vi "Launch He Line.vi"(8 "error in (no error)":errorcluster, 9 "Interlock Chain":refnum<class "Interlock Chain.lvclass">, 11 "cRIO-CO2 in":refnum<class "cRIO-CO2.lvclass">) -> (0 "error out":errorcluster, 3 "cRIO-CO2 out":refnum<class "cRIO-CO2.lvclass">)   [LabVIEW 2015, in "cRIO-Carbondioxide.lvlib" / "cRIO-CO2.lvlib" / "cRIO-CO2.lvclass"]
uses:
  cRIO-CO2.lvclass
  Interlocks/Interlock Chain/Interlock Chain.lvclass
  He Line/He Line.lvclass
  <vilib>/ActorFramework/Actor/Actor.lvclass
  Valve/Valve.lvclass
  Valve/Action.ctl
  cRIO-CO2.lvclass/cRIO-CO2.ctl
  <vilib>/ActorFramework/Message Enqueuer/Message Enqueuer.lvclass
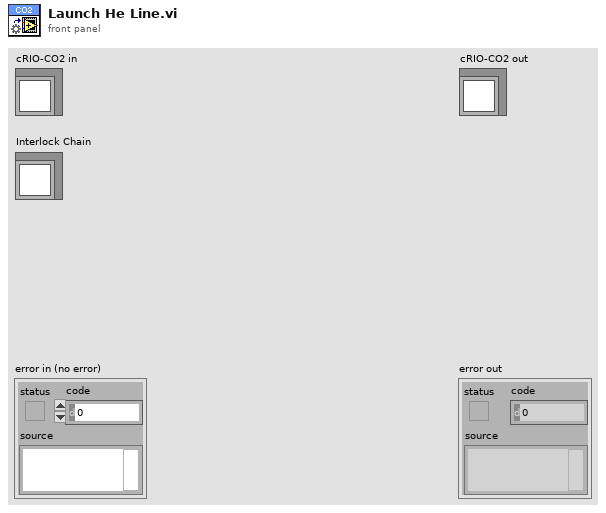
[diagram p1: front panel]
types:
  T1 = typedef "Action.ctl" = enum16{"Open", "Close", "None"}
  T2 = typedef "Dedicated Enqueuers.ctl" = cluster{"Freezers":cluster{"Syringe":refnum<class "Message Enqueuer.lvclass">, "Tank 1":refnum<class "Message Enqueuer.lvclass">, "Tank 2":refnum<class "Message Enqueuer.lvclass">, "Tank 3":refnum<class "Message Enqueuer.lvclass">, "Tank 4":refnum<class "Message Enqueuer.lvclass">}, "Heaters":cluster{"Syringe":refnum<class "Message Enqueuer.lvclass">, "Piston":refnum<class "Message Enqueuer.lvclass">}, "Blowers":cluster{"Tank 1":refnum<class "Message Enqueuer.lvclass">, "Tank 2":refnum<class "Message Enqueuer.lvclass">, "Tank 3":refnum<class "Message Enqueuer.lvclass">, "Tank 4":refnum<class "Message Enqueuer.lvclass">, "Syringe":refnum<class "Message Enqueuer.lvclass">}, "Sample Line":refnum<class "Message Enqueuer.lvclass">, "Storage Line":refnum<class "Message Enqueuer.lvclass">, "Transfer Line":refnum<class "Message Enqueuer.lvclass">, "Syringe Stepper":refnum<class "Message Enqueuer.lvclass">, "Syringe Line":refnum<class "Message Enqueuer.lvclass">, "Capillary Line":refnum<class "Message Enqueuer.lvclass">, "Preparation Line":refnum<class "Message Enqueuer.lvclass">, "Turbo":refnum<class "Message Enqueuer.lvclass">, "Vacuum":refnum<class "Message Enqueuer.lvclass">, "He Line":refnum<class "Message Enqueuer.lvclass">, "Cylinder":refnum<class "Message Enqueuer.lvclass">}
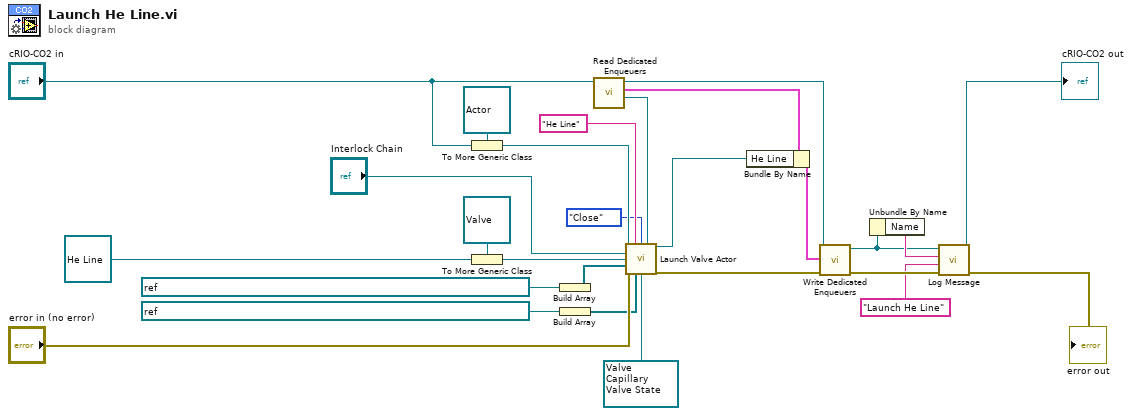
[diagram p0: block diagram]
diagram:
  n1 = To More Generic Class(target class=refnum<class "Actor.lvclass"> refnum ("Caller Actor in"), reference="cRIO-CO2 in") -> (generic class reference=w22:refnum<class "Actor.lvclass">)
  n2 = To More Generic Class(target class=refnum<class "Valve.lvclass"> refnum ("Valve in"), reference=refnum<class "He Line.lvclass"> refnum ("cRIO-Carbondioxide.lvlib:CO2-Actor.lvlib:He Line.lvclass")) -> (generic class reference=w23:refnum<class "Valve.lvclass">)
  n3 = Build Array(refnum<k21> "ni.var.io://crio-carbondioxide/Mod2/He Line Valve DV318" ("SHV")) -> (w7:refnum<k21>[])
  n4 = Build Array(refnum<k21> "ni.var.psp://crio-carbondioxide/AMS Gas SHV/Valves/He Line" ("SHV")) -> (w17:refnum<k21>[])
  n5 = call "Read Dedicated Enqueuers.vi"("cRIO-CO2 in"="cRIO-CO2 in") -> ("Qs.DedicatedEnQrs"=w13:refnum<queue>, "Dedicated Enqueuers"=w12:T2, "cRIO-CO2 out"=w11:refnum<class "cRIO-CO2.lvclass">)  [unwired: 7 in, 1 out]
  n6 = call "Launch Valve Actor.vi"("Caller Actor in"=w22, "Name"="He Line", "Start Action (Open)"=Action."Close", "DedicatedEnQrs"=w13, "Interlock Chain"="Interlock Chain", "Valve in"=w23, "SHV Aliases"=w7, "error in (no error)"="error in (no error)", "SHV"=w17, "StateQ"=refnum<queue> refnum) -> ("Caller-To-Actor Enqueuer"=w9:refnum<class "Message Enqueuer.lvclass">, "error out"=w15:errorcluster)  [unwired: 4 in]
  n7 = Bundle By Name(cluster=w12, "He Line"=w9) -> (w10:T2)
  n8 = call "Write Dedicated Enqueuers.vi"("error in (no error)"=w15, "Dedicated Enqueuers"=w10, "cRIO-CO2 in"=w11) -> ("error out"=w5:errorcluster, "cRIO-CO2 out"=w3:refnum<class "cRIO-CO2.lvclass">)  [unwired: 7 in]
  n9 = Unbundle By Name(w3) -> ("Name"=w6:string)
  n10 = call "Log Message.vi"("error in (no error)"=w5, "String"="Launch He Line", "Source Name"=w6, "cRIO-CO2 in"=w3) -> ("error out"=→"error out":errorcluster, "cRIO-CO2 out"=→"cRIO-CO2 out":refnum<class "cRIO-CO2.lvclass">)  [unwired: 6 in]
